vi "Prepare Paths For Expiration Check.vi"(0 "Vector Path Group in":refnum<class "Vector 18GHz Path Group.lvclass">, 5 "TSM Context":T1, 11 "error in (no error)":errorcluster) -> (4 "Vector Path Group out":refnum<class "Vector 18GHz Path Group.lvclass">, 15 "error out":errorcluster)   [LabVIEW 2023, in "RFFixtureCharact.RFPM.lvlib" / "Vector 18GHz Path Group.lvclass"]
uses:
  Vector 18GHz Path Group.lvclass
  C:/srd-semi-rfcal-software/AuxTools/STSRFFixtureCharactUtility/Source/Code Modules/Common/Base Classes/Path Group/Path Group.lvclass
  <vilib>/NI_TestStand_SemiconductorModule/NI_TestStand_Semiconductor_Module.lvlibp/PinMap/General/SemiconductorModuleContext.ctl
  Paths/Vector Path/Vector 18GHz Path.lvclass
  C:/srd-semi-rfcal-software/AuxTools/STSRFFixtureCharactUtility/Source/Code Modules/Common/Base Classes/Path/Path.lvclass
  Charact Result Accessor/Vector/Vector Charact Result Accessor.lvclass
  C:/srd-semi-rfcal-software/AuxTools/STSRFFixtureCharactUtility/Source/Code Modules/Fixture/RFPM/Charact Result Accessor/Base/Charact Result Accessor.lvclass
  C:/srd-semi-rfcal-software/AuxTools/STSRFFixtureCharactUtility/Source/Code Modules/Common/Result Accessor/Result Accessor.lvclass
  <vilib>/NI_TestStand_SemiconductorModule/NI_TestStand_Semiconductor_Module.lvlibp/PinMap/RF/RFPM/PinToNIRFPMSessionsWithPaths.vi
  Common/Base Classes/Path/Path.lvclass
  Common/Result Accessor/Result Accessor.lvclass
  <vilib>/NI_TestStand_SemiconductorModule/NI_TestStand_Semiconductor_Module.lvlibp
  Common/Base Classes/Path Group/Path Group.lvclass
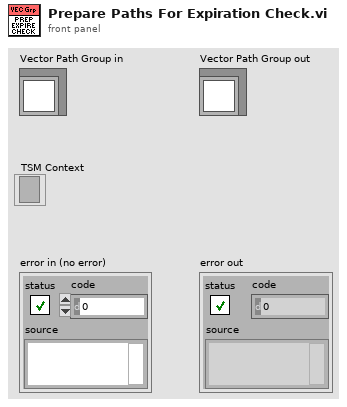
[diagram p1: front panel]
types:
  T1 = typedef "NI_TestStand_Semiconductor_Module.lvlibp/SemiconductorModuleContext.ctl" = refnum<k7>
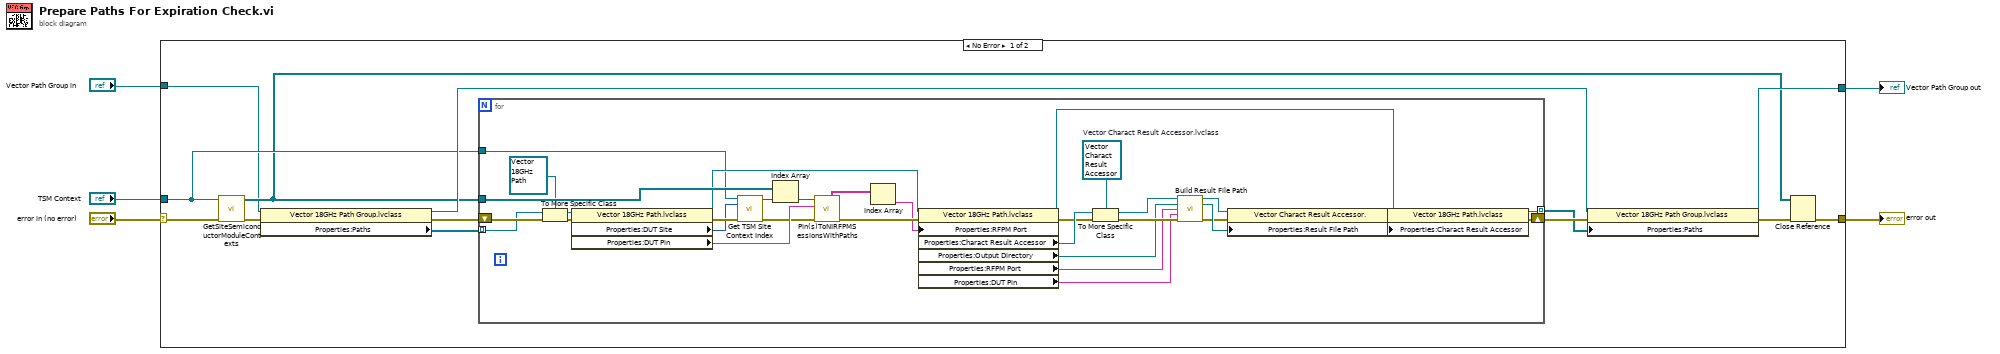
[diagram p0: block diagram]
diagram:
  n1 = case shown="No Error" "error in (no error)" {
    selector: "error in (no error)" -> [w11 w53]
    tunnel: "TSM Context" -> [w13 _]
    tunnel: "Vector Path Group in" -> [w6 w52]
    tunnel: [w14 w53] -> w2
    tunnel: [w15 w52] -> w1
    frame No Error {
      n2 = call <vilib>:"GetSiteSemiconductorModuleContexts.vi"("error in (no error)"=w11, "Semiconductor Module Context"=w13) -> ("error out"=w17:errorcluster, "Site Semiconductor Module Contexts"=w9:T1[])  [unwired: 8 in]
      n3 = property class="Vector 18GHz Path Group.lvclass"(reference=w6, error in=w17) -> (reference out=w16:refnum<class "Vector 18GHz Path Group.lvclass">, error out=w18:errorcluster, "Properties:Paths"=w10:refnum<class "Path.lvclass">[])
      n4 = for {
        tunnel: w9 -> [w51]
        tunnel: w10 -> [w45] mode=indexing
        tunnel: [w29] -> w7 mode=indexing
        tunnel: w13 -> [w39]
        shift-right: [w30] -> w8
        shift-left: w18 -> [w47]
        w34 = refnum<class "Vector Charact Result Accessor.lvclass"> refnum  # Vector Charact Result Accessor.lvclass
        n5 = To More Specific Class(target class=refnum<class "Vector 18GHz Path.lvclass"> refnum ("STS Vector Fixture Charact.lvlib:Vector Path.lvclass"), reference=w45, error in=w47) -> (specific class reference=w44:refnum<class "Vector 18GHz Path.lvclass">, error out=w46:errorcluster)
        n6 = property class="Vector 18GHz Path.lvclass"(reference=w44, error in=w46) -> (reference out=w48:refnum<class "Vector 18GHz Path.lvclass">, error out=w49:errorcluster, "Properties:DUT Site"=w41:i32, "Properties:DUT Pin"=w43:string)
        n7 = call "Get TSM Site Context Index.vi"("Semiconductor Module Context"=w39, "Site Number"=w41, "error in (no error)"=w49) -> ("index of Site TSM Context"=w40:i32, "error out"=w42:errorcluster)  [unwired: 11 in]
        n8 = Index Array(array=w51, index=w40) -> (element=w50:T1)
        n9 = call-poly <vilib>:"Pin(s)ToNIRFPMSessionsWithPaths.vi"("error in (no error)"=w42, "Pin"=w43, "Semiconductor Module Context"=w50) -> ("error out"=w38:errorcluster, "Ports List"=w37:string[])  [unwired: 3 in, 4 out]
        n10 = Index Array(array=w37) -> (element=w36:string)  [unwired: 1 in]
        n11 = property class="Vector 18GHz Path.lvclass"(reference=w48, error in=w38, "Properties:RFPM Port"=w36) -> (reference out=w28:refnum<class "Vector 18GHz Path.lvclass">, error out=w27:errorcluster, "Properties:Charact Result Accessor"=w31:refnum<class "Result Accessor.lvclass">, "Properties:Output Directory"=w21:path, "Properties:RFPM Port"=w20:string, "Properties:DUT Pin"=w19:string)
        n12 = To More Specific Class(target class=w34, reference=w31, error in=w27) -> (specific class reference=w25:refnum<class "Vector Charact Result Accessor.lvclass">, error out=w23:errorcluster)
        n13 = call-dynamic "Build Result File Path.vi"("Vector Charact Result Accessor in"=w25, "Output Directory"=w21, "Port 1"=w20, "Port 2"=w19, "error in"=w23) -> ("Vector Charact Result Accessor out"=w24:refnum<class "Vector Charact Result Accessor.lvclass">, "Result File Path"=w26:path, "error out"=w22:errorcluster)  [unwired: 8 in]
        n14 = property class="Vector Charact Result Accessor."(reference=w24, error in=w22, "Properties:Result File Path"=w26) -> (reference out=w32:refnum<class "Vector Charact Result Accessor.lvclass">, error out=w33:errorcluster)
        n15 = property class="Vector 18GHz Path.lvclass"(reference=w28, error in=w33, "Properties:Charact Result Accessor"=w32) -> (reference out=w29:refnum<class "Vector 18GHz Path.lvclass">, error out=w30:errorcluster)
      }
      n16 = property class="Vector 18GHz Path Group.lvclass"(reference=w16, error in=w8, "Properties:Paths"=w7) -> (reference out=w15:refnum<class "Vector 18GHz Path Group.lvclass">, error out=w12:errorcluster)
      n17 = Close Reference(reference=w9, error in (no error)=w12) -> (error out=w14:errorcluster)
    }
    frame Error {
    }
  }
  "error out" <- w2
  "Vector Path Group out" <- w1
